vi "PH_Beckhoff.ProcPeriodic.vi"(0 "i ref in":refnum<vi>, 3 "ms timeout (10000)":i32=10000, 5 "error in (no error)":errorcluster) -> (14 "i ref out":refnum<vi>, 17 "timed out":bool, 19 "error out":errorcluster)   [LabVIEW 2014, in "PH_Beckhoff.lvlib"]
doc: "This method serves to periodically do things like reading values from the HW. Methods that should be executed periodically should be called from THIS methode. Add code here."
uses:
  PH_Beckhoff.lvlib
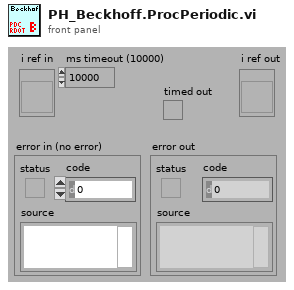
[diagram p1: front panel]
types:
  T1 = typedef "PH_Beckhoff.lvlib/PH_Beckhoff.i attribute.ctl" = cluster{"GUI Refs":T2, "operation?":bool, "Default Prdc Interval":i32, "Connection":T3, "AMS Net ID":T4, "Klemmencluster: # of":T5, "Values":T6, "IP":string, "Description":string, "configured?":bool, "Change Manager":cluster{"Detemination wanted?":bool, "Values changed at":cluster{"Sonderklemmen Inputs":i32[], "Analog Inputs":i32[], "Analog Outputs":i32[], "Digital Inputs":i32[], "Digital Outputs":i32[]}}, "Difference to handle an analog input as change":u32}
  T2 = typedef "PH_Beckhoff.lvlib/PH_Beckhoff.GUI Refs.ctl" = cluster{"ADS Error":refnum<vi>, "Values":refnum<vi>, "configured?":refnum<vi>, "Connection":refnum<vi>, "IP":refnum<vi>, "Prdc Int [ms]":refnum<vi>}
  T3 = typedef "PH_Beckhoff.lvlib/PH_Beckhoff.Connectivity.ctl" = cluster{"DLL?":bool, "Port?":bool, "Client?":bool, "Ping?":bool, "unsuccessful Pings":u32}
  T4 = typedef "Beckhoff - Driver np.lvlib/Beckhoff Access.ctl" = cluster{"DLL path":path, "AMS Net ID":cluster{"1st # of IP":u8, "2nd # of IP":u8, "3rd # of IP":u8, "4th # of IP":u8, "In Port":u8, "Out Port":u8}}
  T5 = typedef "Beckhoff - Driver np.lvlib/Klemmendeclarer.ctl" = cluster{"Offset due to Sonderklemms":u32, "analog Inputs":u32, "analog Outputs":u32, "digital Input Bits":u32, "digital Output Bits":u32}
  T6 = typedef "PH_Beckhoff.lvlib/PH_Beckhoff.Values.ctl" = cluster{"Sonderklemmen Inputs":T7, "Analog Inputs":T8, "Analog Outputs":T10, "Digital Inputs":T11, "Digital Outputs":T12}
  T7 = typedef "PH_Beckhoff.lvlib/PH_Beckhoff.Sonderklemmen Inputs.ctl" = cluster{"Total Length":u32, "Name":string, "Value":u64, "Quality":bool, "Service ID":i32, "Offset":u32, "Length":u32}[]
  T8 = typedef "PH_Beckhoff.lvlib/PH_Beckhoff.Analog Inputs.ctl" = cluster{"Name":string, "Value":u32, "Quality":bool, "Service ID":i32, "Sca Type":T9}[]
  T9 = typedef "PH_Beckhoff.lvlib/PH_Beckhoff.Scaling Type.ctl" = enum16{"none", "0 ... 15 Bit -> 0 ... 5", "0 ... 15 Bit -> 0 ... 10", "0 ... 15 Bit -> 0 ... 25", "0 ... 15 Bit -> 4 ... 20", "0 ... 15 Bit -> 0 ... 1", "0 ... 15 Bit -> 0 ... 20000", "0 ... 15 Bit -> 0 ... 24000"}
  T10 = typedef "PH_Beckhoff.lvlib/PH_Beckhoff.Analog Outputs.ctl" = cluster{"Name":string, "Value":u32, "Quality":bool, "Wanted Value":u32, "Service ID":i32, "Sca Type":T9}[]
  T11 = typedef "PH_Beckhoff.lvlib/PH_Beckhoff.Digital Inputs.ctl" = cluster{"Name":string, "Value":bool, "Quality":bool, "Service ID":i32, "inverted?":bool}[]
  T12 = typedef "PH_Beckhoff.lvlib/PH_Beckhoff.Digital Outputs.ctl" = cluster{"Name":string, "Value":bool, "Quality":bool, "Wanted Value":bool, "Service ID":i32, "inverted?":bool}[]
  T13 = cluster{"Sonderklemmen Inputs":i32[], "Analog Inputs":i32[], "Analog Outputs":i32[], "Digital Inputs":i32[], "Digital Outputs":i32[]}
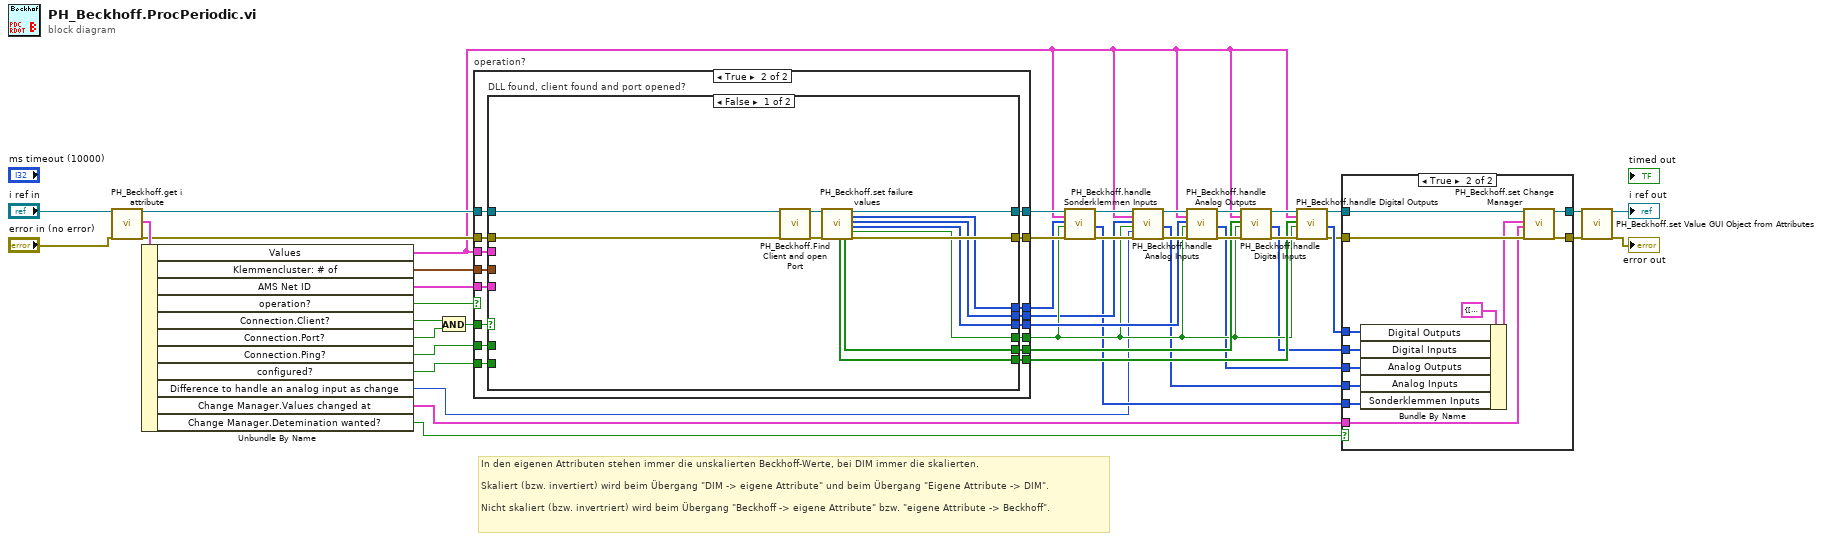
[diagram p0: block diagram]
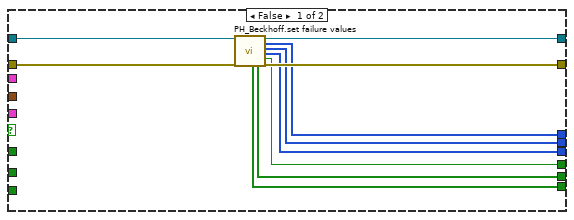
[diagram p3: hidden frame]
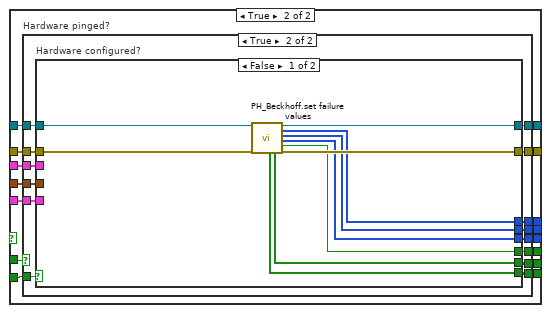
[diagram p4: hidden frame]
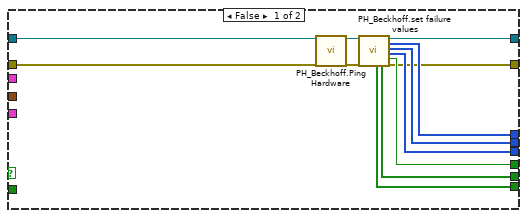
[diagram p5: hidden frame]
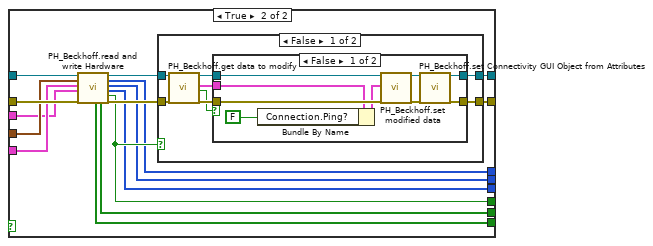
[diagram p6: hidden frame]
diagram:
  # "In den eigenen Attributen stehen immer die unskalierten Beckhoff-Werte, bei DIM immer die skalierten.\n\nSkaliert (bzw. invertiert) wird beim Übergang \"DIM -> eigene Attribute\" und beim Übergang \"Eigene Attribute -> DIM\".\n\nNicht skaliert (bzw. invertriert) wird beim Übergang \"Beckhoff -> eigene Attribute\" bzw. \"eigene Attribute -> Beckhoff\"."
  n1 = call "PH_Beckhoff.get i attribute.vi"("i ref in"="i ref in", "error in (no error)"="error in (no error)") -> ("i ref out"=w40:refnum<vi>, "i attribute"=w42:T1, "error out"=w39:errorcluster)  [unwired: 15 in]
  n2 = Unbundle By Name(w42) -> ("Values"=w19:T6, "Klemmencluster: # of"=w17:T5, "AMS Net ID"=w16:T4, "operation?"=w15:bool, "Connection.Client?"=w38:bool, "Connection.Port?"=w37:bool, "Connection.Ping?"=w20:bool, "configured?"=w18:bool, "Difference to handle an analog input as change"=w1:u32, "Change Manager.Values changed at"=w9:T13, "Change Manager.Detemination wanted?"=w2:bool)
  n3 = And(x=w38, y=w37) -> (x .and. y?=w41:bool)
  n4 = case "operation?" shown="True" w15 {
    tunnel: [w51 w68] -> w27
    tunnel: [w53 w67] -> w28
    tunnel: w39 -> [w52 w70]
    tunnel: w40 -> [w54 w69]
    tunnel: w20 -> [_ w66]
    tunnel: w41 -> [_ w65]
    tunnel: w16 -> [_ w64]
    tunnel: w17 -> [_ w63]
    tunnel: [w50 w62] -> w23
    tunnel: [w45 w61] -> w26
    tunnel: [w46 w60] -> w25
    tunnel: [w49 w59] -> w24
    tunnel: [w48 w58] -> w22
    tunnel: [w47 w57] -> w21
    tunnel: w19 -> [_ w56]
    tunnel: w18 -> [_ w55]
    frame False {
      n5 = call "PH_Beckhoff.set failure values.vi"("i ref in"=w54, "error in"=w52) -> ("Failure Values Digital Outputs"=w45:bool[], "Failure Values Digital Inputs"=w46:bool[], "i ref out"=w53:refnum<vi>, "Failure Values Sonderklemmen Inputs"=w47:u32[], "Failure Values Analog Inputs"=w48:u32[], "Failure Values Analog Outputs"=w49:u32[], "Read and write successful?"=w50:bool, "error out"=w51:errorcluster)  [unwired: 10 in]
    }
    frame True {
      n6 = case "DLL found, client found and port opened?" shown="False" w65 {
        tunnel: w70 -> [w81 w96]
        tunnel: w69 -> [w82 w97]
        tunnel: [w77 w91] -> w68
        tunnel: [w79 w92] -> w67
        tunnel: w66 -> [_ w95]
        tunnel: w64 -> [_ w94]
        tunnel: w63 -> [_ w93]
        tunnel: [w73 w90] -> w62
        tunnel: [w71 w89] -> w61
        tunnel: [w72 w88] -> w60
        tunnel: [w74 w87] -> w59
        tunnel: [w75 w86] -> w58
        tunnel: [w76 w85] -> w57
        tunnel: w56 -> [_ w84]
        tunnel: w55 -> [_ w83]
        frame False {
          n7 = call "PH_Beckhoff.Find Client and open Port.vi"("i ref in"=w82, "error in"=w81) -> ("i ref out"=w80:refnum<vi>, "error out"=w78:errorcluster)  [unwired: 16 in]
          n8 = call "PH_Beckhoff.set failure values.vi"("i ref in"=w80, "error in"=w78) -> ("Failure Values Digital Outputs"=w71:bool[], "Failure Values Digital Inputs"=w72:bool[], "i ref out"=w79:refnum<vi>, "Failure Values Sonderklemmen Inputs"=w76:u32[], "Failure Values Analog Inputs"=w75:u32[], "Failure Values Analog Outputs"=w74:u32[], "Read and write successful?"=w73:bool, "error out"=w77:errorcluster)  [unwired: 10 in]
        }
        frame True {
          n9 = case "Hardware pinged?" shown="True" w95 {
            tunnel: w97 -> [w109 w120]
            tunnel: w96 -> [w108 w121]
            tunnel: [w98 w122] -> w91
            tunnel: [w100 w123] -> w92
            tunnel: w94 -> [_ w112]
            tunnel: w93 -> [_ w113]
            tunnel: [w107 w119] -> w90
            tunnel: [w106 w114] -> w89
            tunnel: [w105 w115] -> w88
            tunnel: [w103 w116] -> w87
            tunnel: [w104 w117] -> w86
            tunnel: [w102 w118] -> w85
            tunnel: w84 -> [_ w111]
            tunnel: w83 -> [_ w110]
            frame False {
              n10 = call "PH_Beckhoff.Ping Hardware.vi"("i ref in"=w109, "error in"=w108) -> ("i ref out"=w101:refnum<vi>, "error out"=w99:errorcluster)  [unwired: 16 in]
              n11 = call "PH_Beckhoff.set failure values.vi"("i ref in"=w101, "error in"=w99) -> ("Failure Values Digital Outputs"=w106:bool[], "Failure Values Digital Inputs"=w105:bool[], "i ref out"=w100:refnum<vi>, "Failure Values Sonderklemmen Inputs"=w102:u32[], "Failure Values Analog Inputs"=w104:u32[], "Failure Values Analog Outputs"=w103:u32[], "Read and write successful?"=w107:bool, "error out"=w98:errorcluster)  [unwired: 10 in]
            }
            frame True {
              n12 = case "Hardware configured?" shown="False" w110 {
                tunnel: [w132 w148] -> w123
                tunnel: [w130 w147] -> w122
                tunnel: w121 -> [w131 w145]
                tunnel: w120 -> [w133 w144]
                tunnel: [w126 w142] -> w119
                tunnel: [w129 w141] -> w118
                tunnel: [w128 w140] -> w117
                tunnel: [w127 w139] -> w116
                tunnel: [w125 w138] -> w115
                tunnel: [w124 w137] -> w114
                tunnel: w113 -> [_ w136]
                tunnel: w112 -> [_ w135]
                tunnel: w111 -> [_ w134]
                frame False {
                  n13 = call "PH_Beckhoff.set failure values.vi"("i ref in"=w133, "error in"=w131) -> ("Failure Values Digital Outputs"=w124:bool[], "Failure Values Digital Inputs"=w125:bool[], "i ref out"=w132:refnum<vi>, "Failure Values Sonderklemmen Inputs"=w129:u32[], "Failure Values Analog Inputs"=w128:u32[], "Failure Values Analog Outputs"=w127:u32[], "Read and write successful?"=w126:bool, "error out"=w130:errorcluster)  [unwired: 10 in]
                }
                frame True {
                  n14 = call "PH_Beckhoff.read and write Hardware.vi"("i ref in"=w144, "Klemmencluster: # of"=w136, "Beckhoff Access"=w135, "Current Values"=w134, "error in"=w145) -> ("Current Digital Output"=w137:bool[], "Current Digital Inputs"=w138:bool[], "i ref out"=w143:refnum<vi>, "Current Sonderklemmen  Inputs"=w141:u64[], "Current Analog Inputs"=w140:u32[], "Current Analog Outputs"=w139:u32[], "Read and write successful?"=w142:bool, "error out"=w146:errorcluster)  [unwired: 7 in]
                  n15 = case shown="False" w142 {
                    tunnel: w146 -> [w156 w169]
                    tunnel: [w150 w169] -> w147
                    tunnel: [w151 w168] -> w148
                    tunnel: w143 -> [w149 w168]
                    frame False {
                      n16 = call "PH_Beckhoff.get data to modify.vi"("i ref in"=w149, "error in (no error)"=w156) -> ("i ref out"=w154:refnum<vi>, "i attribute"=w153:T1, "timed out"=w152:bool, "error out"=w155:errorcluster)  [unwired: 14 in]
                      n17 = case shown="False" w152 {
                        tunnel: w155 -> [w165 w166]
                        tunnel: [w157 w166] -> w150
                        tunnel: w154 -> [w164 w167]
                        tunnel: [w159 w167] -> w151
                        tunnel: w153 -> [w163 _]
                        frame False {
                          n18 = Bundle By Name(cluster=w163, "Connection.Ping?"=FALSE) -> (w162:T1)
                          n19 = call "PH_Beckhoff.set modified data.vi"("i ref in"=w164, "i attribute"=w162, "error in (no error)"=w165) -> ("i ref out"=w160:refnum<vi>, "error out"=w158:errorcluster)  [unwired: 15 in]
                          n20 = call "PH_Beckhoff.set Connectivity GUI Object from Attributes.vi"("i ref in"=w160, "error in"=w158) -> ("i ref out"=w159:refnum<vi>, "error out"=w157:errorcluster)  [unwired: 16 in]
                        }
                        frame True {
                        }
                      }
                    }
                    frame True {
                    }
                  }
                }
              }
            }
          }
        }
      }
    }
  }
  n21 = call "PH_Beckhoff.handle Sonderklemmen Inputs.vi"("i ref in"=w28, "Old Values"=w19, "Current Sonderklemmen Inputs"=w21, "Quality"=w23, "error in"=w27) -> ("i ref out"=w30:refnum<vi>, "#s of changed Sonderklemmen Inputs"=w14:i32[], "error out"=w29:errorcluster)  [unwired: 12 in]
  n22 = call "PH_Beckhoff.handle Analog Inputs.vi"("i ref in"=w30, "Old Values"=w19, "Current Analog Inputs"=w22, "Quality"=w23, "Difference to handle an analog input as change"=w1, "error in"=w29) -> ("i ref out"=w35:refnum<vi>, "#s of changed analog Inputs"=w13:i32[], "error out"=w33:errorcluster)  [unwired: 11 in]
  n23 = call "PH_Beckhoff.handle Analog Outputs.vi"("i ref in"=w35, "Old Values"=w19, "Current Analog Outputs"=w24, "Quality"=w23, "error in"=w33) -> ("i ref out"=w36:refnum<vi>, "#s of changed analog Outputs"=w12:i32[], "error out"=w32:errorcluster)  [unwired: 12 in]
  n24 = call "PH_Beckhoff.handle Digital Inputs.vi"("i ref in"=w36, "Old Values"=w19, "Current Digital Inputs"=w25, "Quality"=w23, "error in"=w32) -> ("i ref out"=w34:refnum<vi>, "#s of changed digital Inputs"=w11:i32[], "error out"=w31:errorcluster)  [unwired: 12 in]
  n25 = call "PH_Beckhoff.handle Digital Outputs.vi"("i ref in"=w34, "Old Values"=w19, "Current Digital Outputs"=w26, "Quality"=w23, "error in"=w31) -> ("i ref out"=w8:refnum<vi>, "#s of changed digital Outputs"=w10:i32[], "error out"=w7:errorcluster)  [unwired: 12 in]
  n26 = case shown="True" w2 {
    tunnel: w14 -> [_ w183]
    tunnel: w13 -> [_ w182]
    tunnel: w12 -> [_ w181]
    tunnel: w11 -> [_ w180]
    tunnel: w10 -> [_ w179]
    tunnel: w9 -> [_ w174]
    tunnel: w8 -> [w171 w178]
    tunnel: w7 -> [w170 w177]
    tunnel: [w171 w176] -> w6
    tunnel: [w170 w175] -> w4
    frame False {
    }
    frame True {
      n27 = Bundle By Name(cluster=T13 {"Sonderklemmen Inputs"=[], "Analog Inputs"=[], "Analog Outputs"=[], "Digital Inputs"=[], "Digital Outputs"=[]} ("Current Value Changes"), "Digital Outputs"=w179, "Digital Inputs"=w180, "Analog Outputs"=w181, "Analog Inputs"=w182, "Sonderklemmen Inputs"=w183) -> (w172:T13)
      n28 = call "PH_Beckhoff.set Change Manager.vi"("i ref in"=w178, "Current Value Changes"=w172, "Old Value Changes"=w174, "error in"=w177) -> ("i ref out"=w176:refnum<vi>, "error out"=w175:errorcluster)  [unwired: 14 in]
    }
  }
  n29 = call "PH_Beckhoff.set Value GUI Object from Attributes.vi"("i ref in"=w6, "error in"=w4) -> ("i ref out"=→"i ref out":refnum<vi>, "error out"=→"error out":errorcluster)  [unwired: 16 in]
